vi "TREE_Read all tems by an giffen path.vi"(8 "error in":errorcluster, 9 "pattern":string, 10 "path to start the search":path, 11 "Tree In":refnum<vi>) -> (0 "error out":errorcluster, 1 "Number of files found":i32, 3 "Tree Out":refnum<vi>)   [LabVIEW 2011]
panel:
  in  "File dialog? (F)":bool
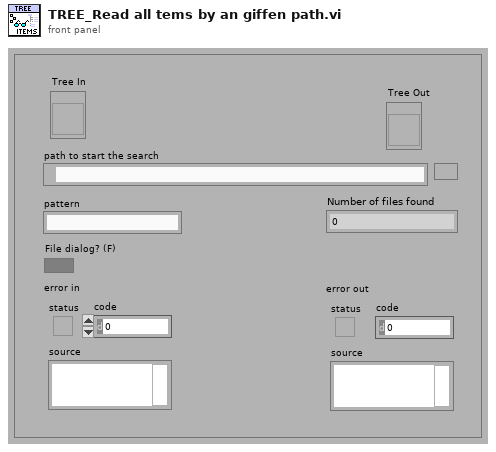
[diagram p1: front panel]
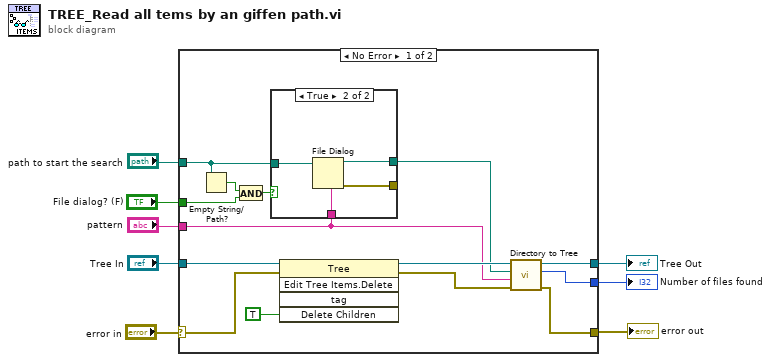
[diagram p0: block diagram]
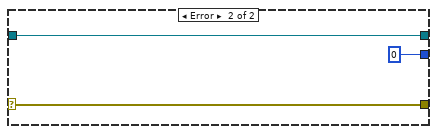
[diagram p3: hidden frame]
diagram:
  n1 = case shown="No Error" "error in" {
    selector: "error in" -> [w9 w30]
    tunnel: "Tree In" -> [w19 w29]
    tunnel: [w18 w29] -> w7
    tunnel: [w17 w30] -> w6
    tunnel: [w16 0 ("Number of files found")] -> w5
    tunnel: "path to start the search" -> [w14 _]
    tunnel: "pattern" -> [w13 _]
    tunnel: "File dialog? (F)" -> [w10 _]
    frame No Error {
      n2 = Empty String/Path?(string/path=w14) -> (empty?=w12:bool)
      n3 = And(x=w12, y=w10) -> (x .and. y?=w11:bool)
      n4 = case shown="True" w11 {
        tunnel: [w23 w26] -> w15
        tunnel: w14 -> [w23 w27]
        tunnel: w13 -> [_ w25]
        tunnel: [_ w24] -> _
        frame False {
        }
        frame True {
          n5 = File Dialog(4:w25, 11:w27) -> (0:w24:errorcluster, 3:w26:path)  [unwired: 5 in, 2 out]
        }
      }
      n6 = invoke on="Invoke Node" class="Tree" method="Edit Tree Items.Delete"(reference=w19, error in=w9, "Delete Children"=TRUE ("Open")) -> (reference out=w21:refnum<vi>, error out=w20:errorcluster)  [unwired: 2 in, 3 out]
      n7 = call <userlib>:"Directory to Tree.vi"("error in"=w20, "Pattern"=w13, "Path to start the search"=w15, "Tree In"=w21) -> ("error out"=w17:errorcluster, "Number of files found"=w16:i32, "Tree Out"=w18:refnum<vi>)  [unwired: 2 in, 1 out]
    }
    frame Error {
    }
  }
  "Tree Out" <- w7
  "error out" <- w6
  "Number of files found" <- w5
